vi "Determine Operating Point.vi"(2 "Tag.lvclass":refnum<class "Tag.lvclass">, 7 "error in (no error)":errorcluster) -> (13 "error out":errorcluster, 14 "OperatingPointA":dbl, 15 "OperatingPointB":dbl, 16 "Heading":dbl, 17 "step size":dbl, 18 "fOperatingPointA":dbl, 19 "fOperatingPointB":dbl)   [LabVIEW 2014, in "Tag.lvclass"]
doc: "This VI is used to determine a Tag's next 'werkpunt' (operating point). Based on it's current and previous position(s) it is able to predict what its next step will be, approximately. Returns 'OperatingPointA' and 'OperatingPointB' which correspond to the x & y coordinates respectively."
uses:
  Tag.lvclass
panel:
  out "TagY":dbl
  out "TagX":dbl
  out "deltaY":dbl
  out "deltaX":dbl
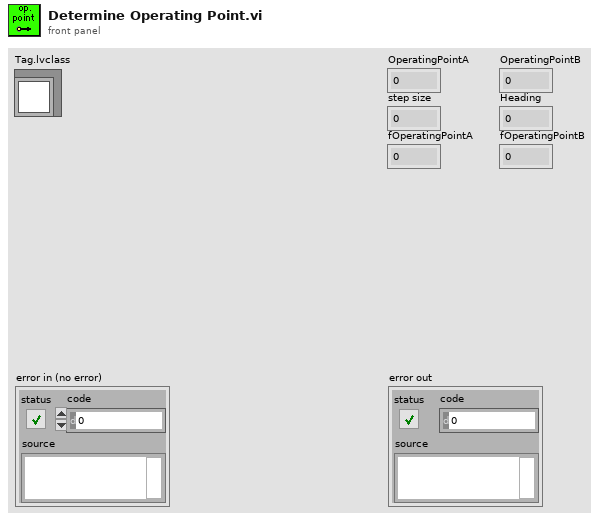
[diagram p1: front panel]
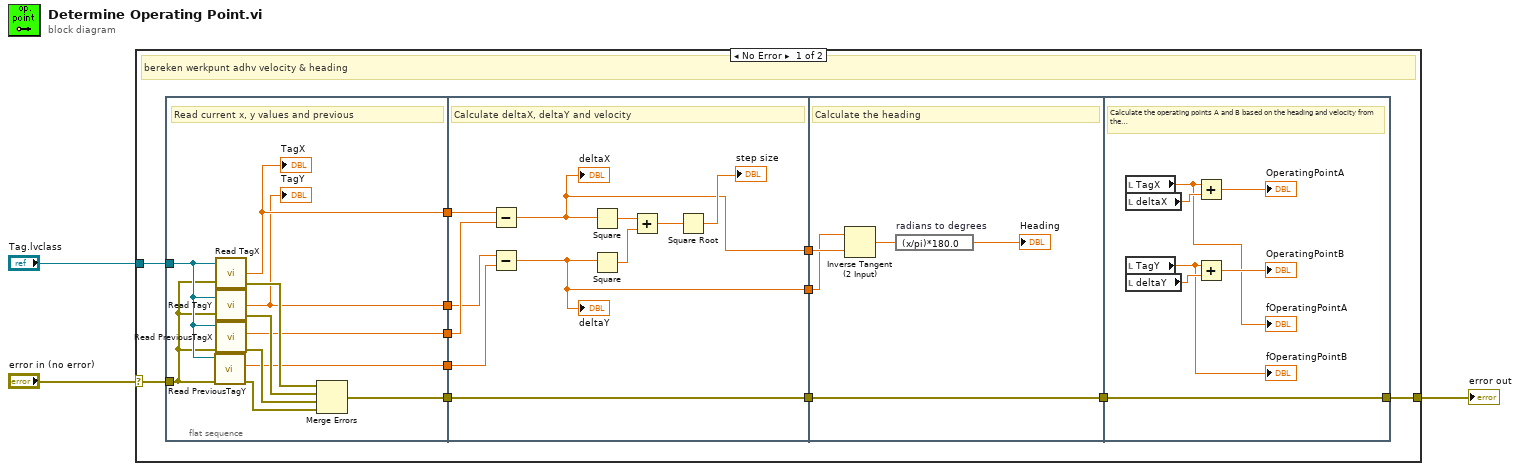
[diagram p0: block diagram]
diagram:
  n1 = case shown="No Error" "error in (no error)" {
    selector: "error in (no error)" -> [w14 w50]
    tunnel: [w13 w50] -> w2
    tunnel: "Tag.lvclass" -> [w15 _]
    frame No Error {
      # "bereken werkpunt adhv velocity & heading"
      n2 = flat-sequence {
        tunnel: w15 -> [w26]
        tunnel: w14 -> [w25]
        tunnel: [w24] -> w12
        tunnel: [w19] -> w10
        tunnel: [w18] -> w9
        tunnel: [w16] -> w8
        tunnel: [w17] -> w7
        tunnel: w12 -> [w37]
        tunnel: [w37] -> w11
        tunnel: w10 -> [w30]
        tunnel: w9 -> [w29]
        tunnel: w8 -> [w27]
        tunnel: w7 -> [w28]
        tunnel: [w32] -> w6
        tunnel: [w31] -> w5
        tunnel: w11 -> [w42]
        tunnel: w6 -> [w39]
        tunnel: w5 -> [w40]
        tunnel: [w42] -> w4
        tunnel: [w49] -> w13
        tunnel: w4 -> [w49]
        frame #0 {
          # "Read current x, y values and previous"
          n3 = call-dynamic "Read PreviousTagY.vi"("error in (no error)"=w25, "Tag in"=w26) -> ("error out"=w23:errorcluster, "PreviousTagY"=w17:dbl)  [unwired: 7 in, 1 out]
          n4 = call-dynamic "Read TagX.vi"("Tag in"=w26, "error in (no error)"=w25) -> ("RealTagX"=w19:dbl, "error out"=w20:errorcluster)  [unwired: 1 out]
          "TagX" <- w19
          n5 = call-dynamic "Read TagY.vi"("Tag in"=w26, "error in (no error)"=w25) -> ("RealTagY"=w16:dbl, "error out"=w21:errorcluster)  [unwired: 1 out]
          "TagY" <- w16
          n6 = call-dynamic "Read PreviousTagX.vi"("error in (no error)"=w25, "Tag in"=w26) -> ("error out"=w22:errorcluster, "PreviousTagX"=w18:dbl)  [unwired: 7 in, 1 out]
          n7 = Merge Errors(w20, w21, w22, w23) -> (w24:errorcluster)
        }
        frame #1 {
          # "Calculate deltaX, deltaY and velocity"
          n8 = Subtract(x=w30, y=w29) -> (x-y=w31:dbl)
          "deltaX" <- w31
          n9 = Subtract(x=w27, y=w28) -> (x-y=w32:dbl)
          "deltaY" <- w32
          n10 = Square(x=w31) -> (x^2=w36:dbl)
          n11 = Square(x=w32) -> (x^2=w35:dbl)
          n12 = Add(x=w36, y=w35) -> (x+y=w34:dbl)
          n13 = Square Root(x=w34) -> (sqrt(x)=→"step size":dbl)
        }
        frame #2 {
          # "Calculate the heading"
          n14 = Inverse Tangent (2 Input)(1:w40, 2:w39) -> (0:w41:dbl)
          n15 = expression code="(x/pi)*180.0" "radians to degrees"(w41) -> (→"Heading":dbl)
        }
        frame #3 {
          # "Calculate the operating points A and B based on the heading and velocity from the \ncurrent x,y coordinates"
          n16 = local read "TagX"() -> (w44:dbl)
          "fOperatingPointA" <- w44
          n17 = local read "deltaX"() -> (w48:dbl)
          n18 = local read "TagY"() -> (w43:dbl)
          "fOperatingPointB" <- w43
          n19 = local read "deltaY"() -> (w47:dbl)
          n20 = Add(x=w44, y=w48) -> (x+y=→"OperatingPointA":dbl)
          n21 = Add(x=w43, y=w47) -> (x+y=→"OperatingPointB":dbl)
        }
      }
    }
    frame Error {
    }
  }
  "error out" <- w2
